vi "Command-CreateDVR.vi"(8 "error in (no error)":errorcluster, 10 "Data":T1, 11 "Engine in":refnum<class "Engine.lvclass">) -> (0 "error out":errorcluster, 3 "Engine out":refnum<class "Engine.lvclass">)   [LabVIEW 2024, in "GLF.lvlib" / "Engine.lvclass"]
uses:
  Engine.lvclass
  Engine.lvclass/Engine.ctl
  IAmGLF/IAmGLF.lvclass
  Command-CreateDVR--cluster.ctl
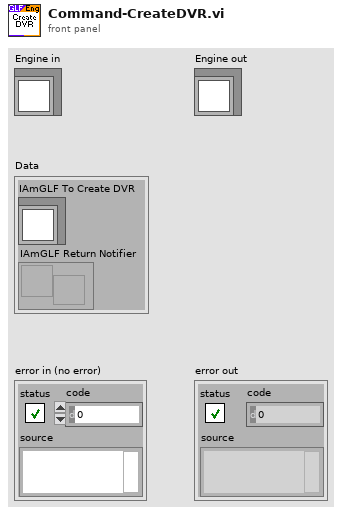
[diagram p1: front panel]
types:
  T1 = typedef "GLF.lvlib/Engine.lvclass/Command-CreateDVR--cluster.ctl" = cluster{"IAmGLF To Create DVR":refnum<class "IAmGLF.lvclass">, "IAmGLF Return Notifier":refnum<notifier>}
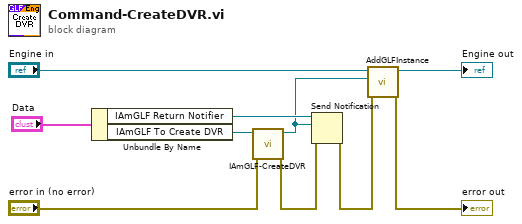
[diagram p0: block diagram]
diagram:
  n1 = Unbundle By Name("Data") -> ("IAmGLF Return Notifier"=w9:refnum<notifier>, "IAmGLF To Create DVR"=w10:refnum<class "IAmGLF.lvclass">)
  n2 = call-dynamic "IAmGLF-CreateDVR.vi"("error in (no error)"="error in (no error)", "IAmGLF in"=w10) -> ("error out"=w3:errorcluster, "IAmGLF out"=w8:refnum<class "IAmGLF.lvclass">)  [unwired: 8 in]
  n3 = Send Notification(notification=w8, notifier=w9, error in (no error)=w3) -> (error out=w2:errorcluster)  [unwired: 1 out]
  n4 = call "AddGLFInstance.vi"("error in (no error)"=w2, "GLF Instance"=w8, "Engine in"="Engine in") -> ("error out"=→"error out":errorcluster, "Engine out"=→"Engine out":refnum<class "Engine.lvclass">)  [unwired: 7 in]
